vi "Load_Info.vi"(8 "error in (no error)":errorcluster, 11 "AB_SourceDistribution in":refnum<class "AB_SourceDistribution.lvclass">) -> (0 "error out":errorcluster, 3 "AB_SourceDistribution out":refnum<class "AB_SourceDistribution.lvclass">)   [LabVIEW 2020, in "AB_SourceDistribution.lvclass"]
uses:
  <vilib>/AppBuilder/AB_Classes/SourceDistribution/AB_SourceDistribution.lvclass
  e:/builds/penguin/labview/branches/2020/dev/dist/vi.lib/AppBuilder/AB_Classes/Build/AB_Build.lvclass
  <vilib>/AppBuilder/AB_Classes/Build/AB_Build.lvclass
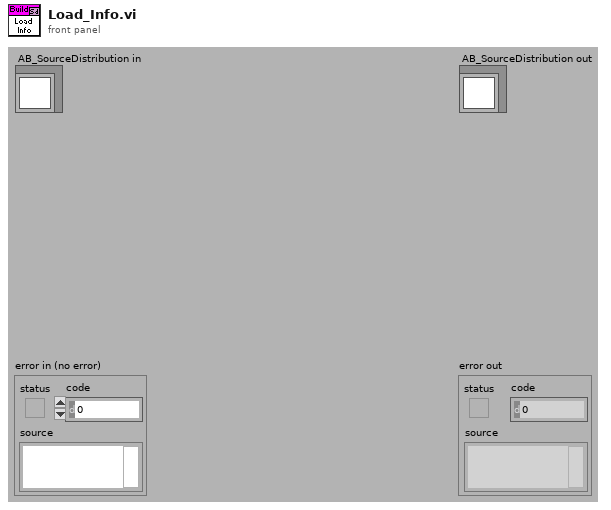
[diagram p1: front panel]
types:
  T1 = typedef "AB_Build.ctl" = cluster{"buildSpecName":string, "buildSpecDescription":string, "destinations":refnum<class "AB_Destination.lvclass">[], "exclusionOption":T2, "defaultLanguage":string, "supportedLanguages":string[], "excludedDirectories":path[], "buildContext":refnum<vi>, "buildObject":T3, "preview":bool, "programatic":bool, "progressBarEvents":T4, "userLog_Path":path, "preActionID":string, "preAction_Path":path, "postActionID":string, "postAction_Path":path, "eng_checkForBrokenVIs?":bool, "eng_verboseLinkerErrors?":bool, "localDest_Path":path, "targetDest_Path":path, "removeVIObject":u16, "cache":refnum<class "PreviewCache.lvclass">, "use cache":bool, "previewCache_ID":string, "buildCache_ID":string, "eng_TempLocalDest_Path":path, "eng_collectDependencies?":bool, "versionInfo":cluster{"buildVersion":cluster{"major":u16, "minor":u16, "patch":u16, "build":u16}, "autoIncrement":bool}, "eng_enableVIChecksums":bool}
  T2 = typedef "AB_Exclusion_Option.ctl" = cluster{"typedefs":bool, "polymorphicVIs":bool, "unusedLibraryItems":bool, "modifyLibraryFile":bool, "edit-timeDependencies":bool, "inlineVIs":bool, "dependent PPLs":bool, "dependent DLLs":bool}
  T3 = typedef "ItemRef.ctl" = u64
  T4 = typedef "provcom_ProgressBar_Events.ctl" = cluster{"newJob":refnum<user-event>, "newItem":refnum<user-event>, "errorMsg":T5, "cancel":refnum<user-event>}
  T5 = typedef "mxLvBuildError.ctl" = refnum<user-event>
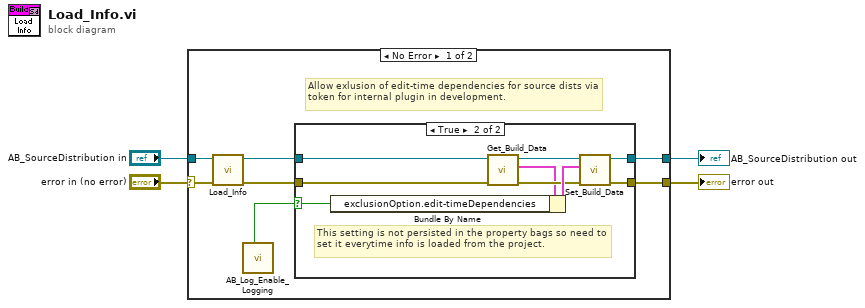
[diagram p0: block diagram]
diagram:
  n1 = case shown="No Error" "error in (no error)" {
    selector: "error in (no error)" -> [w10 w23]
    tunnel: [w9 w23] -> w4
    tunnel: [w8 w24] -> w3
    tunnel: "AB_SourceDistribution in" -> [w11 w24]
    frame No Error {
      # "Allow exlusion of edit-time dependencies for source dists via token for internal plugin in development."
      n2 = call-parent "Load_Info.vi"("error in (no error)"=w10, "AB_Build in"=w11) -> ("error out"=w5:errorcluster, "AB_Build out"=w6:refnum<class "AB_SourceDistribution.lvclass">)  [unwired: 8 in]
      n3 = call <vilib>:"AB_Log_Enable_Logging.vi"() -> ("sdist_exclude_edittime"=w7:bool)  [unwired: 4 in, 7 out]
      n4 = case shown="True" w7 {
        selector: w7 -> [_ w14]
        tunnel: w6 -> [w13 w19]
        tunnel: w5 -> [w12 w17]
        tunnel: [w12 w22] -> w9
        tunnel: [w13 w20] -> w8
        frame False {
        }
        frame True {
          # "This setting is not persisted in the property bags so need to set it everytime info is loaded from the project."
          n5 = call <vilib>:"Get_Build_Data.vi"("error in (no error)"=w17, "Class in"=w19) -> ("error out"=w16:errorcluster, "data"=w15:T1, "Class out"=w18:refnum<class "AB_SourceDistribution.lvclass">)  [unwired: 7 out]
          n6 = Bundle By Name(cluster=w15, "exclusionOption.edit-timeDependencies"=w14) -> (w21:T1)
          n7 = call <vilib>:"Set_Build_Data.vi"("error in (no error)"=w16, "data"=w21, "Class in"=w18) -> ("error out"=w22:errorcluster, "Class out"=w20:refnum<class "AB_SourceDistribution.lvclass">)  [unwired: 7 out]
        }
      }
    }
    frame Error {
    }
  }
  "error out" <- w4
  "AB_SourceDistribution out" <- w3
